vi "niusrprios DUC (Multi-Channel).vi"(0 "data in":T1[](array[typedef]), 1 "reset":bool, 5 "enabled":bool[](array[boolean]), 9 "input valid":bool, 11 "DUC Parameters":T2[](array[typedef]) {"frequency shift" format="%#.48g"}) -> (4 "I data out":i16[](array[numeric]), 6 "Q data out":i16[](array[numeric]), 10 "output valid":bool, 13 "dsp reset done":bool, 14 "ready for input":bool, 15 "number of overflows":u64[](array[numeric]))   [LabVIEW 2015]
doc: "Digital upconverter (DUC) for two channels which can be extended to more channels. Implemented with FPGA-based DSP.\n\n<B>Input Parameters</B>\n\n<B>data in</B> is the I and Q data to be upconverted along with overflow information.\n\n<B>enabled</B> specifies which streams are enabled.\n\n<B>input valid</B> specifies when 'data in' is valid.\n\n<B>DUC Parameters</B> are the upconversion parameters utilized by the DSP chain.\n\n<B>reset</B> the DSP upconversion signal chain.\n\n<B>Output Parameters</B>\n\n<B>dsp reset done</B> indicates that the DSP upconversion signal chain completed reset.\n\n<B>ready for input</B> is a flow control signal that indicates whether the DUC is ready to accept new data.\n\n<B>I data out</B> is the in phase component of upconverted data to be transmitted.\n\n<B>Q data out</B> is the quadrature phase component of upconverted data to be transmitted.\n\n<B>output valid</B> specifies when 'data out' is valid.\n\n<B>number of overflows</B> is the number of times the DSP chain overflowed on fixed point conversion of 'data in'."
uses:
  niusrprios DUC Parameters.ctl
  <instrlib>/_niInstr/DSP/v1/Shared/Public/IQ Impairments.ctl
  <instrlib>/_niInstr/DSP/v1/Shared/Public/IQ Gain.ctl
  <instrlib>/_niInstr/DSP/v1/Shared/Public/IQ Data.ctl
  <instrlib>/_niInstr/DSP/v1/Shared/niInstr DSP v1 Shared.lvlib
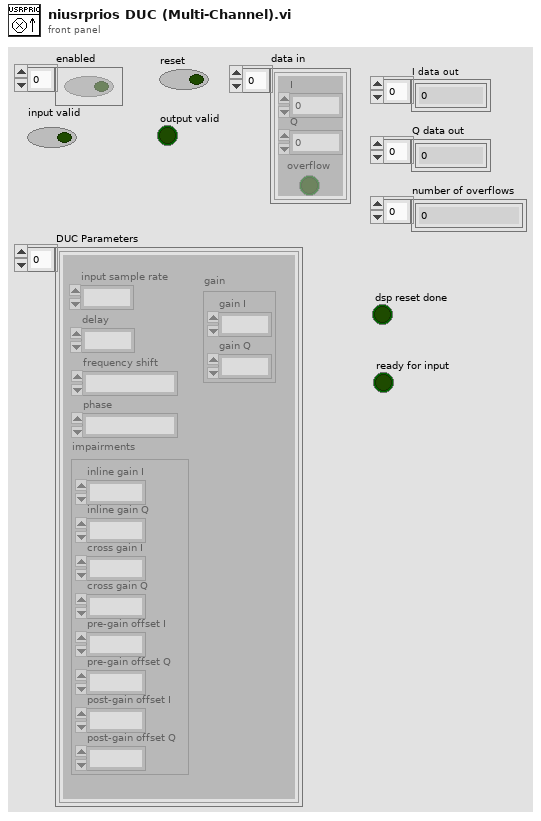
[diagram p1: front panel]
types:
  T1 = typedef "niInstr DSP v1 Shared.lvlib/IQ Data.ctl" = cluster{"I":fxp<+/-,18,1>, "Q":fxp<+/-,18,1>, "overflow":bool}
  T2 = typedef "niusrprios DUC Parameters.ctl" = cluster{"frequency shift":fxp<+/-,48,0>, "impairments":T3, "phase":fxp<+/-,21,0>, "input sample rate":fxp<+,48,1>, "gain":T4, "delay":fxp<+/-,18,0>}
  T3 = typedef "niInstr DSP v1 Shared.lvlib/IQ Impairments.ctl" = cluster{"inline gain I":fxp<+/-,18,1>, "inline gain Q":fxp<+/-,18,1>, "cross gain I":fxp<+/-,18,1>, "cross gain Q":fxp<+/-,18,1>, "pre-gain offset I":fxp<+/-,18,1>, "pre-gain offset Q":fxp<+/-,18,1>, "post-gain offset I":fxp<+/-,18,1>, "post-gain offset Q":fxp<+/-,18,1>}
  T4 = typedef "niInstr DSP v1 Shared.lvlib/IQ Gain.ctl" = cluster{"gain I":fxp<+/-,24,3>, "gain Q":fxp<+/-,24,3>}
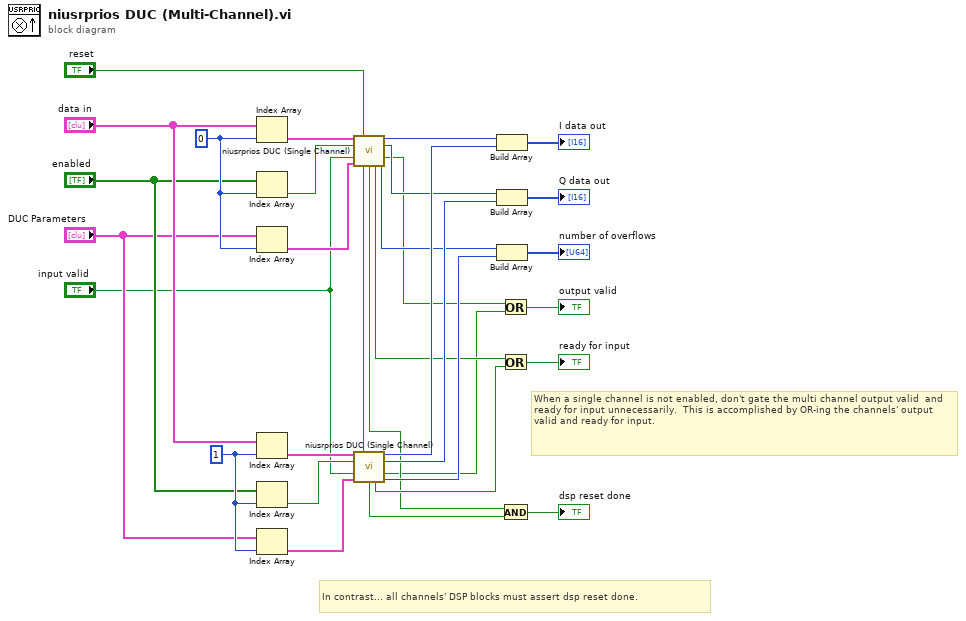
[diagram p0: block diagram]
diagram:
  w30 = 1 ("index")
  w31 = 0 ("index")
  # "When a single channel is not enabled, don't gate the multi channel output valid  and ready for input unnecessarily.  This is accomplished by OR-ing the channels' output valid and ready for input."
  # "In contrast... all channels' DSP blocks must assert dsp reset done."
  n1 = Index Array(array="data in", index=w31) -> (element=w28:T1)
  n2 = Index Array(array="enabled", index=w31) -> (element=w4:bool)
  n3 = Index Array(array="DUC Parameters", index=w31) -> (element=w27:T2)
  n4 = Index Array(array="data in", index=w30) -> (element=w24:T1)
  n5 = Index Array(array="enabled", index=w30) -> (element=w23:bool)
  n6 = Index Array(array="DUC Parameters", index=w30) -> (element=w22:T2)
  n7 = call "niusrprios DUC (Single Channel).vi"("data in"=w28, "reset"="reset", "enabled"=w4, "input valid"="input valid", "DUC Parameters"=w27) -> ("I data out"=w20:i16, "Q data out"=w17:i16, "output valid"=w2:bool, "dsp reset done"=w5:bool, "ready for input"=w10:bool, "number of overflows"=w14:u64)  [unwired: 5 in]
  n8 = call "niusrprios DUC (Single Channel).vi"("data in"=w24, "reset"="reset", "enabled"=w23, "input valid"="input valid", "DUC Parameters"=w22) -> ("I data out"=w18:i16, "Q data out"=w16:i16, "output valid"=w1:bool, "dsp reset done"=w7:bool, "ready for input"=w9:bool, "number of overflows"=w13:u64)  [unwired: 5 in]
  n9 = Build Array(w20, w18) -> (→"I data out":i16[])
  n10 = Build Array(w17, w16) -> (→"Q data out":i16[])
  n11 = Build Array(w14, w13) -> (→"number of overflows":u64[])
  n12 = Or(x=w2, y=w1) -> (x .or. y?=→"output valid":bool)
  n13 = Or(x=w10, y=w9) -> (x .or. y?=→"ready for input":bool)
  n14 = And(x=w5, y=w7) -> (x .and. y?=→"dsp reset done":bool)
